vi "Example Simple.vi"() -> ()   [LabVIEW 2010]
uses:
  C:/tf/play/labview/Tinkerforge.dll
  Tinkerforge.dll
panel:
  out "z (G)":sgl
  out "y (G)":sgl
  out "x (G)":sgl
  in  "uid":string="abc"
  in  "port":i32=4223
  in  "host":string="localhost"
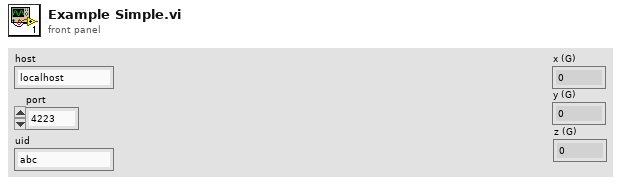
[diagram p1: front panel]
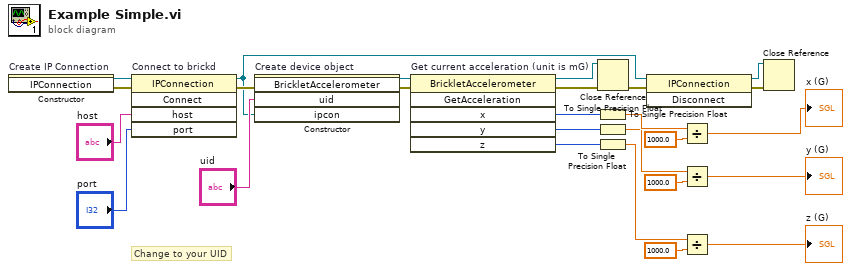
[diagram p0: block diagram]
diagram:
  # "Change to your UID"
  n1 = constructor on="Create IP Connection" class="IPConnection"() -> (reference out=w26:refnum<k24>, error out=w13:errorcluster)  [unwired: 3 in, 1 out]
  n2 = invoke on="Connect to brickd" class="IPConnection" method="Connect"(reference=w26, error in=w13, "host"="host", "port"="port") -> (reference out=w15:refnum<k24>, error out=w22:errorcluster)  [unwired: 1 in, 3 out]
  n3 = constructor on="Create device object" class="BrickletAccelerometer"(error in=w22, "uid"="uid", "ipcon"=w15) -> (reference out=w20:refnum<k24>, error out=w21:errorcluster)  [unwired: 2 in, 3 out]
  n4 = invoke on="Get current acceleration (unit is mG)" class="BrickletAccelerometer" method="GetAcceleration"(reference=w20, error in=w21) -> (reference out=w18:refnum<k24>, error out=w19:errorcluster, "x"=w11:i16, "y"=w1:i16, "z"=w4:i16)  [unwired: 4 in, 1 out]
  n5 = Close Reference(reference=w18, error in (no error)=w19) -> (error out=w17:errorcluster)
  n6 = To Single Precision Float(number=w11) -> (single precision float=w10:sgl)
  n7 = To Single Precision Float(number=w1) -> (single precision float=w7:sgl)
  n8 = To Single Precision Float(number=w4) -> (single precision float=w5:sgl)
  n9 = invoke class="IPConnection" method="Disconnect"(reference=w15, error in=w17) -> (reference out=w14:refnum<k24>, error out=w16:errorcluster)  [unwired: 1 in, 1 out]
  n10 = Divide(x=w10, y=sgl 1000.0) -> (x/y=→"x (G)":sgl)
  n11 = Divide(x=w7, y=sgl 1000.0) -> (x/y=→"y (G)":sgl)
  n12 = Divide(x=w5, y=sgl 1000.0) -> (x/y=→"z (G)":sgl)
  n13 = Close Reference(reference=w14, error in (no error)=w16) -> ()  [unwired: 1 out]
